vi "DeleteServers.vi"(3 "Delete servers on close":bool=TRUE) -> ()   [LabVIEW 2012]
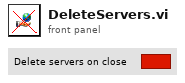
[diagram p1: front panel]
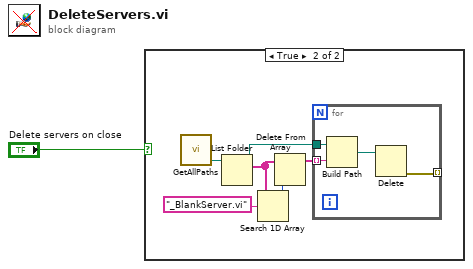
[diagram p0: block diagram]
diagram:
  n1 = case shown="True" "Delete servers on close" {
    frame False {
    }
    frame True {
      n2 = call <userlib>:"GetAllPaths.vi"() -> ("Server Folder"=w2:path)  [unwired: 1 in, 2 out]
      n3 = List Folder(path=w2) -> (path out=w6:path, filenames=w4:string[])  [unwired: 3 in, 2 out]
      n4 = Search 1D Array(1D array=w4, element="_BlankServer.vi") -> (index of element=w5:i32)  [unwired: 1 in]
      n5 = Delete From Array(array=w4, index=w5) -> (array with subset deleted=w7:string[])  [unwired: 1 in, 1 out]
      n6 = for {
        tunnel: w6 -> [w10]
        tunnel: w7 -> [w9] mode=indexing
        tunnel: [w8] -> _ mode=indexing
        n7 = Build Path(base path=w10, name or relative path=w9) -> (appended path=w11:path)
        n8 = Delete(path (use dialog)=w11) -> (error out=w8:errorcluster)  [unwired: 4 in, 2 out]
      }
    }
  }
